vi "Dispose.vi"(8 "error in":errorcluster, 11 "ChicagoStyleClamPizza":refnum<class "ChicagoStyleClamPizza.lvclass">) -> (0 "error out":errorcluster)   [LabVIEW 2020, in "FactoryMethod.lvlib" / "PizzaFactoryMethod.lvlib" / "ChicagoStyleClamPizza.lvclass"]
uses:
  ChicagoStyleClamPizza.lvclass
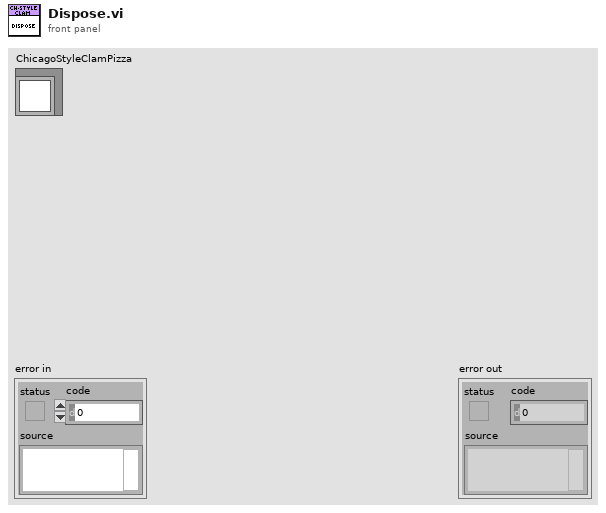
[diagram p1: front panel]
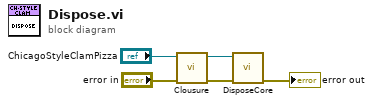
[diagram p0: block diagram]
diagram:
  n1 = call-dynamic "Clousure.vi"("error in"="error in", "ChicagoStyleClamPizza"="ChicagoStyleClamPizza") -> ("error out"=w3:errorcluster, "ChicagoStyleClamPizza"=w4:refnum<class "ChicagoStyleClamPizza.lvclass">)  [unwired: 8 in]
  n2 = call-dynamic "DisposeCore.vi"("error in (no error)"=w3, "ChicagoStyleClamPizza"=w4) -> ("error out"=→"error out":errorcluster)  [unwired: 8 in, 1 out]
